vi "ChangeLight.vi"(0 "object in":refnum<class "YellowState.lvclass">, 5 "Error In":errorcluster) -> (14 "object out":refnum<class "State.lvclass">, 19 "Error Out":errorcluster)   [LabVIEW 2024, in "YellowState.lvclass"]
uses:
  YellowState.lvclass
  State_interface/State.lvclass
  GreenState_class/GreenState.lvclass
  C:/Users/burakkorkmaz/Desktop/Leveling/labview-desing-patterns/State Pattern/State_interface/State.lvclass
  YellowState.lvclass/YellowState.ctl
panel:
  # "Connector Pane"
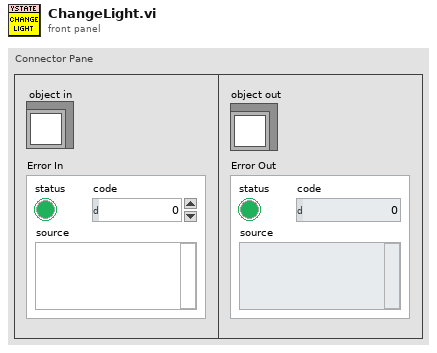
[diagram p1: front panel]
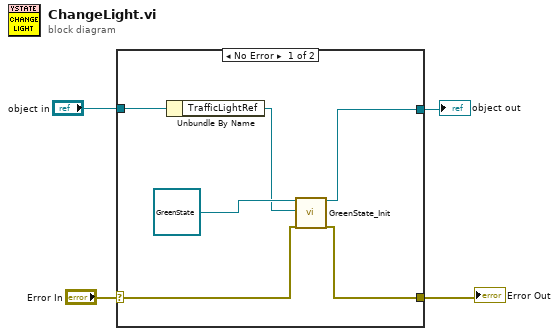
[diagram p0: block diagram]
diagram:
  n1 = case shown="No Error" "Error In" {
    selector: "Error In" -> [w6 w11]
    tunnel: [w8 w11] -> w3
    tunnel: "object in" -> [w10 _]
    tunnel: [w5 _] -> w1
    frame No Error {
      n2 = Unbundle By Name(w10) -> ("TrafficLightRef"=w7:refnum<class "TrafficLight.lvclass">)
      n3 = call "GreenState_Init.vi"("object in"=refnum<class "GreenState.lvclass"> refnum ("GreenState"), "TrafficLight"=w7, "Error In"=w6) -> ("object out"=w5:refnum<class "GreenState.lvclass">, "Error Out"=w8:errorcluster)  [unwired: 15 in]
    }
    frame Error {
    }
  }
  "Error Out" <- w3
  "object out" <- w1
